vi "Unlock Setpoint Write Protection.vi"(0 "Session Handle":T1, 11 "error in (no error)":errorcluster) -> (4 "Session Handle Out":T1, 15 "error out":errorcluster)   [LabVIEW 2015, in "Peltier.lvclass"]
uses:
  Peltier.lvclass
  Typedefs/Session Handle.ctl
  PAS/PAS.lvclass
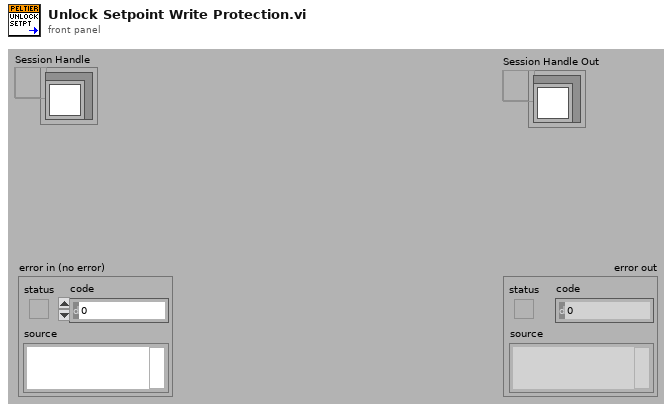
[diagram p1: front panel]
types:
  T1 = typedef "Peltier.lvclass/Session Handle.ctl" = refnum<data-value>
  T2 = typedef "XNET Frame CAN.ctl" = cluster{"timestamp":timestamp, "payload":u8[], "identifier":u32, "type":T3, "extended?":bool, "echo?":bool}
  T3 = typedef "XNET Frame Type CAN.ctl" = u8
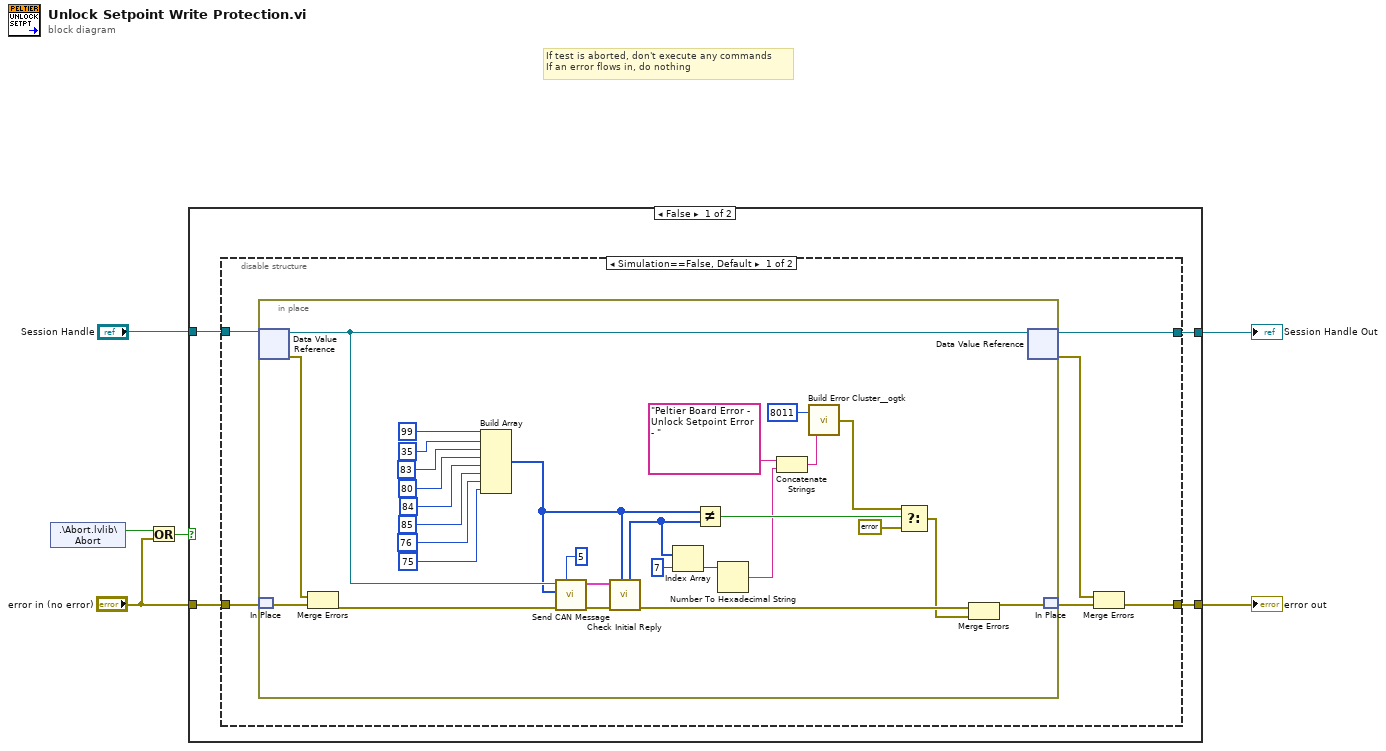
[diagram p0: block diagram]
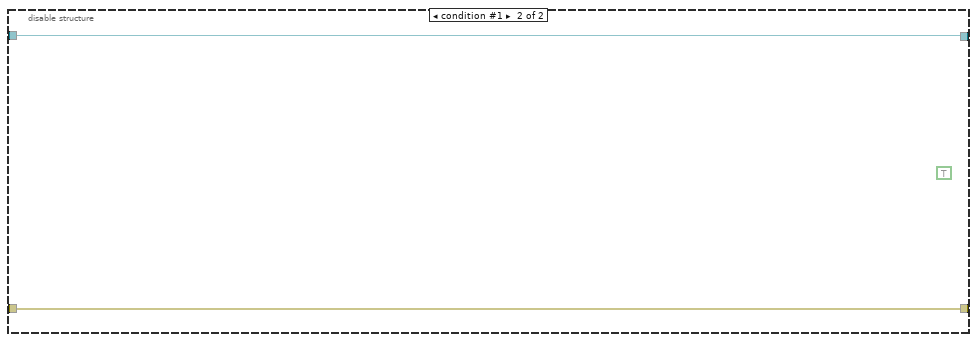
[diagram p2: hidden frame]
diagram:
  # "If test is aborted, don't execute any commands\nIf an error flows in, do nothing"
  n1 = shared-variable ".\\Abort.lvlib\\Abort"() -> (w5:bool)  [unwired: 1 in, 1 out]
  n2 = Or(x=w5, y="error in (no error)") -> (x .or. y?=w3:bool)
  n3 = case shown="False" w3 {
    tunnel: [w10 w49] -> w1
    tunnel: [w9 w48] -> w6
    tunnel: "Session Handle" -> [w8 w49]
    tunnel: "error in (no error)" -> [w7 w48]
    frame False {
      n4 = disable-structure shown="Simulation==False, Default" {
        disable-tunnel: [w16 w47] -> w10
        disable-tunnel: [w13 w46] -> w9
        disable-tunnel: w8 -> [w12 w47]
        disable-tunnel: w7 -> [w11 w46]
        frame condition #0 (active) {
          n5 = in-place {
            n6 = in-place-dvr #1(w12) -> (w36:refnum<class "Peltier.lvclass">, w44:errorcluster)
            n7 = in-place-match #2(w11) -> (w43:errorcluster)
            n8 = Merge Errors(w44, w43) -> (w42:errorcluster)
            n9 = Build Array(u8 99 ("new element/subarray"), u8 35 ("new element/subarray"), u8 83 ("new element/subarray"), u8 80 ("new element/subarray"), u8 84 ("new element/subarray"), u8 85 ("new element/subarray"), u8 76 ("new element/subarray"), u8 75 ("new element/subarray")) -> (w35:u8[])
            n10 = call "Send CAN Message.vi"("Number of Retries"=5, "error in (no error)"=w42, "payload"=w35, "Peltier In"=w36) -> ("error out"=w19:errorcluster, "Reply"=w40:T2[])  [unwired: 5 in, 1 out]
            n11 = call "Check Initial Reply.vi"("Write Message"=w35, "error in (no error)"=w19, "Reply"=w40) -> ("error out"=w18:errorcluster, "Whole Payload"=w33:u8[])  [unwired: 5 in, 2 out]
            n12 = Index Array(array=w33, index=7) -> (element=w31:u8)
            n13 = Not Equal?(x=w35, y=w33) -> (x != y?=w34:bool)
            n14 = Number To Hexadecimal String(2:w31) -> (0:w29:string)  [unwired: 1 in]
            n15 = Concatenate Strings("Peltier Board Error - Unlock Setpoint Error - " ("string"), w29) -> (w28:string)
            n16 = call <userlib>:"Build Error Cluster__ogtk.vi"("String to Prepend to source (\"\")"=w28, "code"=8011) -> ("error out"=w38:errorcluster)
            n17 = Select(t=w38, s=w34, f=errorcluster {"status"=FALSE, "code"=0, "source"=""}) -> (s? t:f=w17:errorcluster)
            n18 = Merge Errors(w18, w17) -> (w45:errorcluster)
            n19 = in-place-dvr #1(w36) -> (w16:T1, w14:errorcluster)
            n20 = in-place-match #2(w45) -> (w15:errorcluster)
          }
          n21 = Merge Errors(w14, w15) -> (w13:errorcluster)
        }
        frame condition #1 {
          (unwired) TRUE
        }
      }
    }
    frame True {
    }
  }
  "error out" <- w6
  "Session Handle Out" <- w1
